vi "ExecuteCommandTemplate.vi"(10 "Params":string[][](array[string]), 11 "Command":string) -> ()   [LabVIEW 2017]
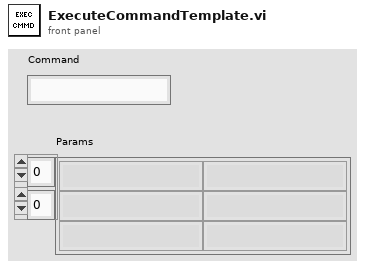
[diagram p1: front panel]
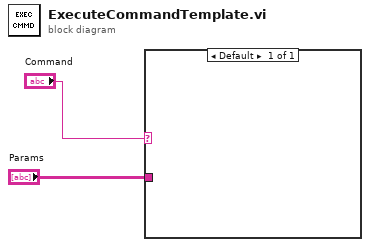
[diagram p0: block diagram]
diagram:
  n1 = case shown="Default" "Command" {
    tunnel: "Params" -> [_]
    frame Default {
    }
  }
